vi "MGI RWA Enque Top Level Data.vi"(5 "Format String (%#_13g)":string, 6 "Conversion":T3, 7 "Read/Write Options":T2={"TS Fmt"="", "Int Fmt"="", "Delimiter"=","}, 8 "Error In":errorcluster, 9 "Anything":variant, 10 "Read String":string, 11 "Data Queue In":refnum<queue>) -> (0 "Error Out":errorcluster, 1 "Read State":T1={"StrToSpecifiedText"=variant, "Specified Data"=variant, "Float Fmt"="%#_13g", "Major Vers"=0, "Options"={"TS Fmt"="", "Int Fmt"="", "Delimiter"=","}}, 2 "Tag to String":variant, 3 "Data Queue Our":refnum<queue>, 4 "Warnings":string)   [LabVIEW 2020]
doc: "Add top level data to processing queue. This VI is called both by String to Anything (To Anything=T) and by Anything to String (To Anything=F). Tag to String and Read State are valid only if To Anything=T.\n\nAuthored by Shawn D. Walpole\nsupport@mooregoodideas.com\nwww.mooregoodideas.com\n\nCopyright (c) 2010, Moore Good Ideas, Inc.\n\nAll rights reserved.\n\nRedistribution and use in source and binary forms, with or without modification, are permitted provided that the following conditions are met:\n\n * Redistributions of source code must retain the above copyright notice, this list of conditions and the following disclaimer.\n * Redistributions in binary form must reproduce the above copyright notice, this list of conditions and the following disclaimer in the documentation and/or other materials provided with the distribution.\n * Neither the name of Moore Good Ideas, Inc. nor the names of its contributors may be used to endorse or promote products derived from this software without specific prior written permission.\n\nTHIS SOFTWARE IS PROVIDED BY THE COPYRIGHT HOLDERS AND CONTRIBUTORS \"AS IS\" AND ANY EXPRESS OR IMPLIED WARRANTIES, INCLUDING, BUT NOT LIMITED TO, THE IMPLIED WARRANTIES OF MERCHANTABILITY AND FITNESS FOR A PARTICULAR PURPOSE ARE DISCLAIMED. IN NO EVENT SHALL THE COPYRIGHT OWNER OR CONTRIBUTORS BE LIABLE FOR ANY DIRECT, INDIRECT, INCIDENTAL, SPECIAL, EXEMPLARY, OR CONSEQUENTIAL DAMAGES (INCLUDING, BUT NOT LIMITED TO, PROCUREMENT OF SUBSTITUTE GOODS OR SERVICES; LOSS OF USE, DATA, OR PROFITS; OR BUSINESS INTERRUPTION) HOWEVER CAUSED AND ON ANY THEORY OF LIABILITY, WHETHER IN CONTRACT, STRICT LIABILITY, OR TORT (INCLUDING NEGLIGENCE OR OTHERWISE) ARISING IN ANY WAY OUT OF THE USE OF THIS SOFTWARE, EVEN IF ADVISED OF THE POSSIBILITY OF SUCH DAMAGE."
uses:
  MGI RWA Options Cluster.ctl
  MGI RWA Convertion Direction Enum.ctl
  MGI RWA Tag Lookup Cluster.ctl
  <vilib>/Utility/VariantDataType/Type.ctl
  <vilib>/Utility/VariantDataType/VariantType.lvlib
  String/MGI Windows Get Regional String/MGI Windows Regional Ring.ctl
  <vilib>/Utility/Data Type/NI_Data Type.lvlib
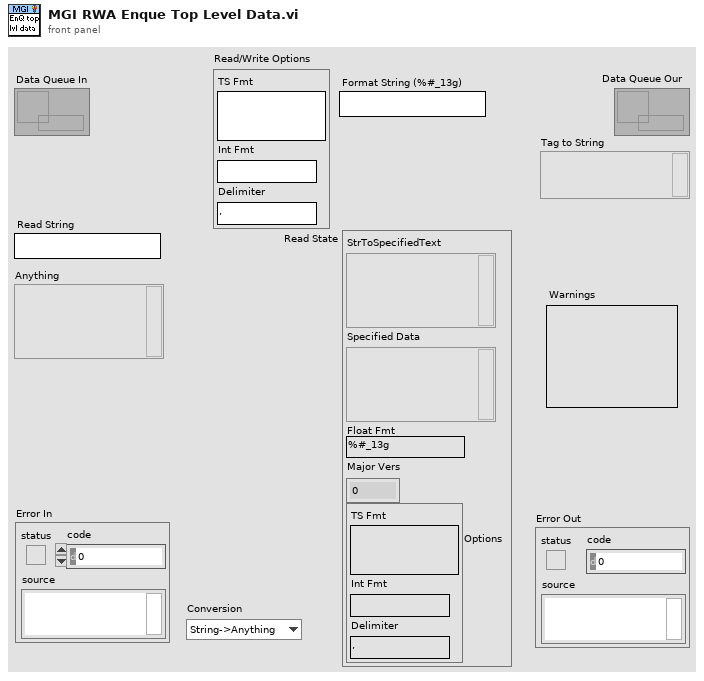
[diagram p1: front panel]
types:
  T1 = typedef "MGI RWA Tag Lookup Cluster.ctl" = cluster{"StrToSpecifiedText":variant, "Specified Data":variant, "Float Fmt":string, "Major Vers":i32, "Options":T2}
  T2 = typedef "MGI RWA Options Cluster.ctl" = cluster{"TS Fmt":string, "Int Fmt":string, "Delimiter":string}
  T3 = typedef "MGI RWA Convertion Direction Enum.ctl" = enum16{"String->Anything", "Anything->String"}
  T4 = typedef "MGI Windows Regional Ring.ctl" = u32
  T5 = typedef "NI_Data Type.lvlib/Data Type.ctl" = enum8{"Invalid Type", "Void", "I8", "I16", "I32", "I64", "U8", "U16", "U32", "U64", "Single Float", "Double Float", "Extended Float", "Single Complex", "Double Complex", "Extended Complex", "Enum U8", "Enum U16", "Enum U32", "Enum U64", "Single Float With Unit", "Double Float With Unit", "Extended Float With Unit", "Single Complex with Unit", "Double Complex with Unit", "Extended Complex with Unit", "Boolean", "String", "Path", "Picture", "Tag", "Array", "Cluster", "Variant", "LV Variant", "Waveform", "Timestamp", "Digital Waveform", "Digital Data", "ExpressData", "Refnum", "External Data", "VI", "Poly VI", "LabVIEW Class Instance", "Fixed Point", "Set Collection", "Map Collection"}
  T6 = typedef "VariantType.lvlib/Type.ctl" = enum8{"Invalid Type", "Void", "I8", "I16", "I32", "I64", "U8", "U16", "U32", "U64", "Single Float", "Double Float", "Extended Float", "Single Complex", "Double Complex", "Extended Complex", "Enum U8", "Enum U16", "Enum U32", "Enum U64", "Single Float With Unit", "Double Float With Unit", "Extended Float With Unit", "Single Complex with Unit", "Double Complex with Unit", "Extended Complex with Unit", "Boolean", "String", "Path", "Picture", "Tag", "Array", "Cluster", "Variant", "LV Variant", "Waveform", "Timestamp", "Digital Waveform", "Digital Data", "ExpressData", "Refnum", "External Data", "VI", "Poly VI", "LabVIEW Class Instance", "Fixed Point"}
  T7 = typedef "NI_Data Type.lvlib/Type Definition Info.ctl" = cluster{"Name":string, "Timestamp":u32}
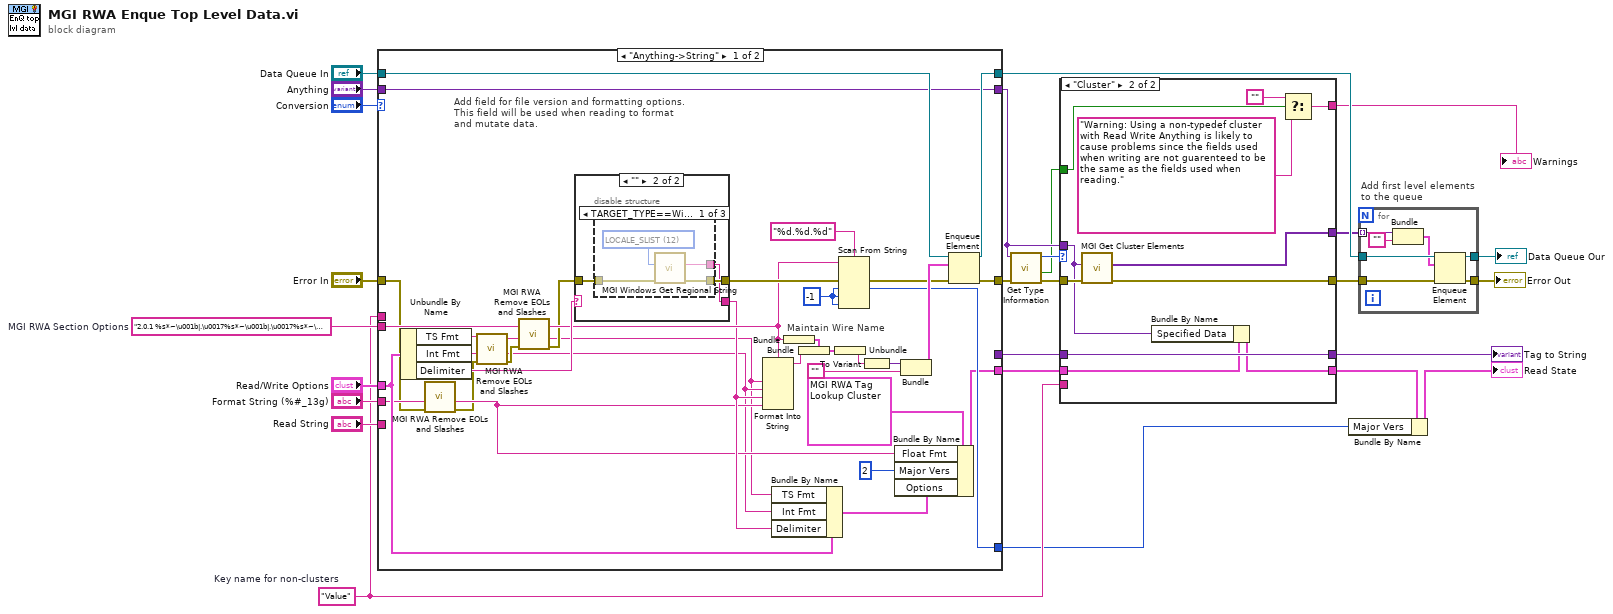
[diagram p0: block diagram]
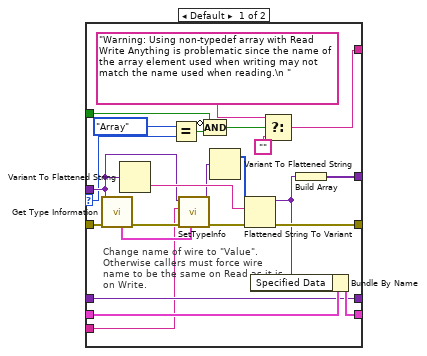
[diagram p2: hidden frame]
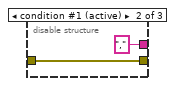
[diagram p4: hidden frame]
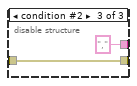
[diagram p5: hidden frame]
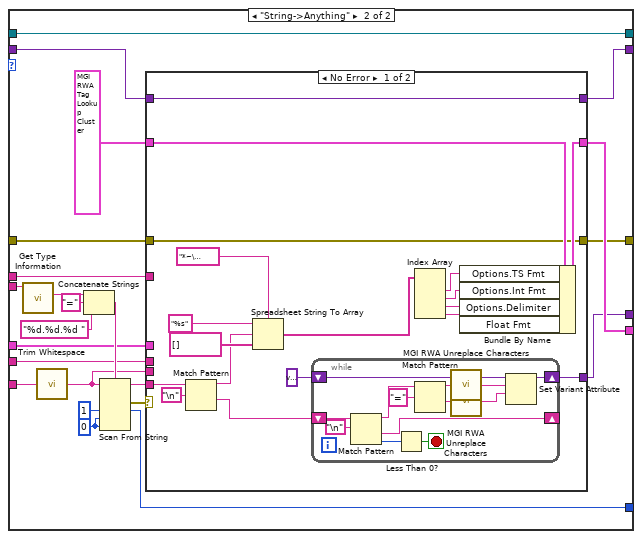
[diagram p6: hidden frame]
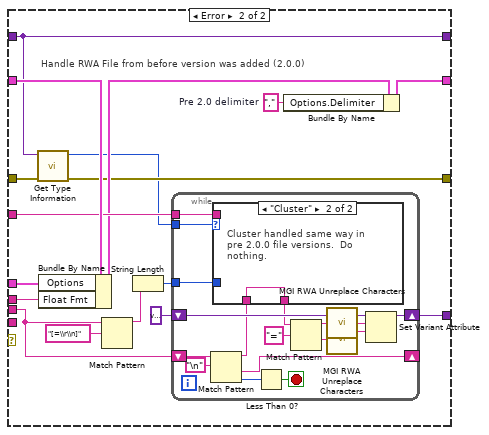
[diagram p7: hidden frame]
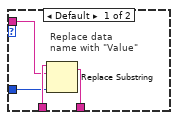
[diagram p8: hidden frame]
diagram:
  w8 = "Value"  # Key name for non-clusters
  w24 = "2.0.1 %s*~\u001b|.\u0017%s*~\u001b|.\u0017%s*~\u001b|.\u0017%s"  # MGI RWA Section Options
  # "Add first level elements\nto the queue"
  n1 = case shown="\"Anything->String\"" "Conversion" {
    tunnel: "Error In" -> [w29 w83]
    tunnel: [w60 w81] -> w13
    tunnel: [w59 w82] -> w26
    tunnel: "Read/Write Options" -> [w40 w86]
    tunnel: w24 -> [w47 w96]
    tunnel: "Data Queue In" -> [w56 w82]
    tunnel: "Format String (%#_13g)" -> [w32 w87]
    tunnel: [w41 w84] -> w10
    tunnel: "Read String" -> [_ w75]
    tunnel: [_ w80] -> w11
    tunnel: [w51 w78] -> w5
    tunnel: w8 -> [_ w79]
    tunnel: "Anything" -> [w48 w77]
    tunnel: [w48 w76] -> w3
    frame "Anything->String" {
      w52 = -1 ("default value 1")
      # "Maintain Wire Name"
      # "Add field for file version and formatting options.  This field will be used when reading to format and mutate data."
      n2 = Unbundle By Name(w40) -> ("TS Fmt"=w34:string, "Int Fmt"=w36:string, "Delimiter"=w49:string)
      n3 = call "MGI RWA Remove EOLs and Slashes.vi"("error in (no error)"=w29, "Format String"=w32) -> ("error out"=w30:errorcluster, "Format String without \\n"=w31:string)  [unwired: 8 in]
      n4 = call "MGI RWA Remove EOLs and Slashes.vi"("error in (no error)"=w30, "Format String"=w36) -> ("error out"=w35:errorcluster, "Format String without \\n"=w28:string)  [unwired: 8 in]
      n5 = call "MGI RWA Remove EOLs and Slashes.vi"("error in (no error)"=w35, "Format String"=w34) -> ("error out"=w33:errorcluster, "Format String without \\n"=w27:string)  [unwired: 8 in]
      n6 = case shown="\"\"" w49 {
        selector: w49 -> [w61 _]
        tunnel: w33 -> [w62 w65]
        tunnel: [w62 w64] -> w50
        tunnel: [w61 w63] -> w39
        frame Default {
        }
        frame "" {
          n7 = disable-structure shown="TARGET_TYPE==Windows" {
            disable-tunnel: [w68 "," ("List Seperator") "," ("List Seperator")] -> w63
            disable-tunnel: w65 -> [w67 w70 w73]
            disable-tunnel: [w66 w70 w73] -> w64
            frame condition #0 {
              w69 = T4 12 items=["LOCALE_ILANGUAGE"=1, "LOCALE_SLANGUAGE"=2, "LOCALE_SABBREVLANGNAME"=3, "LOCALE_SNATIVELANGNAME"=4, "LOCALE_ICOUNTRY"=5, "LOCALE_SCOUNTRY"=6, "LOCALE_SABBREVCTRYNAME"=7, "LOCALE_SNATIVECTRYNAME"=8, "LOCALE_IDEFAULTLANGUAGE"=9, "LOCALE_IDEFAULTCOUNTRY"=10, "LOCALE_IDEFAULTCODEPAGE"=11, "LOCALE_SLIST"=12, "LOCALE_IMEASURE"=13, "LOCALE_SDECIMAL"=14, "LOCALE_STHOUSAND"=15, "LOCALE_SGROUPING"=16, "LOCALE_IDIGITS"=17, "LOCALE_ILZERO"=18, "LOCALE_SNATIVEDIGITS"=19, "LOCALE_SCURRENCY"=20, "LOCALE_SINTLSYMBOL"=21, "LOCALE_SMONDECIMALSEP"=22, "LOCALE_SMONTHOUSANDSEP"=23, "LOCALE_SMONGROUPING"=24, "LOCALE_ICURRDIGITS"=25, "LOCALE_IINTLCURRDIGITS"=26, "LOCALE_ICURRENCY"=27, "LOCALE_INEGCURR"=28, "LOCALE_SDATE"=29, "LOCALE_STIME"=30, "LOCALE_SSHORTDATE"=31, "LOCALE_SLONGDATE"=32, "LOCALE_IDATE"=33, "LOCALE_ILDATE"=34, "LOCALE_ITIME"=35, "LOCALE_ICENTURY"=36, "LOCALE_ITLZERO"=37, "LOCALE_IDAYLZERO"=38, "LOCALE_IMONLZERO"=39, "LOCALE_S1159"=40, "LOCALE_S2359"=41, "LOCALE_SDAYNAME1"=42, "LOCALE_SDAYNAME2"=43, "LOCALE_SDAYNAME3"=44, "LOCALE_SDAYNAME4"=45, "LOCALE_SDAYNAME5"=46, "LOCALE_SDAYNAME6"=47, "LOCALE_SDAYNAME7"=48, "LOCALE_SABBREVDAYNAME1"=49, "LOCALE_SABBREVDAYNAME2"=51, "LOCALE_SABBREVDAYNAME3"=52, "LOCALE_SABBREVDAYNAME4"=53, "LOCALE_SABBREVDAYNAME5"=54, "LOCALE_SABBREVDAYNAME6"=55, "LOCALE_SABBREVDAYNAME7"=56, "LOCALE_SMONTHNAME1"=57, "LOCALE_SMONTHNAME2"=58, "LOCALE_SMONTHNAME3"=59, "LOCALE_SMONTHNAME4"=60, "LOCALE_SMONTHNAME5"=61, "LOCALE_SMONTHNAME6"=62, "LOCALE_SMONTHNAME7"=63, "LOCALE_SMONTHNAME8"=64, "LOCALE_SMONTHNAME9"=65, "LOCALE_SMONTHNAME10"=66, "LOCALE_SMONTHNAME11"=67, "LOCALE_SMONTHNAME12"=68, "LOCALE_SABBREVMONTHNAME1"=69, "LOCALE_SABBREVMONTHNAME2"=70, "LOCALE_SABBREVMONTHNAME3"=71, "LOCALE_SABBREVMONTHNAME4"=72, "LOCALE_SABBREVMONTHNAME5"=73, "LOCALE_SABBREVMONTHNAME6"=74, "LOCALE_SABBREVMONTHNAME7"=75, "LOCALE_SABBREVMONTHNAME8"=76, "LOCALE_SABBREVMONTHNAME9"=77, "LOCALE_SABBREVMONTHNAME10"=78, "LOCALE_SABBREVMONTHNAME11"=79, "LOCALE_SABBREVMONTHNAME12"=80, "LOCALE_SENGLANGUAGE"=4097, "LOCALE_SENGCOUNTRY"=4098, "LOCALE_STIMEFORMAT"=4099, "LOCALE_SABBREVMONTHNAME13"=4111] ("Regional Item")
              n8 = call "MGI Windows Get Regional String.vi"("error in (no error)"=w67, "Regional Item"=w69) -> ("error out"=w66:errorcluster, "List Seperator"=w68:string)  [unwired: 8 in]
            }
            frame condition #1 (active) {
            }
            frame condition #2 {
            }
          }
        }
      }
      n9 = Format Into String(format string=w47, w27, w28, w39, w31) -> (resulting string=w46:string)  [unwired: 2 in, 1 out]
      n10 = Bundle By Name(cluster=w40, "TS Fmt"=w27, "Int Fmt"=w28, "Delimiter"=w39) -> (w38:T2)
      n11 = Bundle("MGI RWA Section Options"=w47) -> (w45:cluster{"MGI RWA Section Options":string})  [unwired: 1 in]
      n12 = Bundle(cluster=w45, "MGI RWA Section Options"=w46) -> (w44:cluster{"MGI RWA Section Options":string})
      n13 = Unbundle(w44) -> ("MGI RWA Section Options"=w43:string)
      n14 = Scan From String(format string="%d.%d.%d", input string=w47, error in=w50, default 1=w52, default 2=w52, default 3=w52) -> (error out=w54:errorcluster, output 1=w51:i32)  [unwired: 3 in, 2 out]
      n15 = To Variant(anything=w43) -> (Variant=w55:variant)
      n16 = Bundle By Name(cluster=T1 {"StrToSpecifiedText"=variant, "Specified Data"=variant, "Float Fmt"="", "Major Vers"=0, "Options"={"TS Fmt"="", "Int Fmt"="", "Delimiter"=""}} ("State In"), "Float Fmt"=w31, "Major Vers"=2, "Options"=w38) -> (w41:T1)
      n17 = Bundle("Variant"=w55, "") -> (w57:cluster{"Variant":variant, string})  [unwired: 1 in]
      n18 = Enqueue Element(queue=w56, element=w57, error in (no error)=w54) -> (queue out=w59:refnum<queue>, error out=w60:errorcluster)  [unwired: 1 in, 1 out]
    }
    frame "String->Anything" {
      w92 = 0 ("default value 1")
      n19 = call <vilib>:"Get Type Information.vi"("variant"=w96) -> ("name"=w95:string)  [unwired: 6 in, 4 out]
      n20 = call <vilib>:"Trim Whitespace.vi"("string"=w75) -> ("trimmed string"=w74:string)  [unwired: 1 in]
      n21 = Concatenate Strings(w95, "=" ("string"), "%d.%d.%d ") -> (w90:string)
      n22 = Scan From String(format string=w90, input string=w74, default 1=1 ("default value 1"), default 2=w92, default 3=w92) -> (remaining string=w88:string, error out=w89:errorcluster, output 1=w78:i32)  [unwired: 4 in, 1 out]
      n23 = case shown="No Error" w89 {
        tunnel: w88 -> [w113 _]
        tunnel: w87 -> [_ w143]
        tunnel: w86 -> [_ w136]
        tunnel: T1 {"StrToSpecifiedText"=variant, "Specified Data"=variant, "Float Fmt"="", "Major Vers"=0, "Options"={"TS Fmt"="", "Int Fmt"="", "Delimiter"=""}} ("State In") -> [w108 w144]
        tunnel: [w107 w134] -> w84
        tunnel: w83 -> [w97 w132]
        tunnel: [w97 w131] -> w81
        tunnel: [w101 w141] -> w80
        tunnel: w79 -> [_ w139]
        tunnel: w77 -> [w98 w130]
        tunnel: [w98 w130] -> w76
        tunnel: w74 -> [_ w128]
        frame No Error {
          n24 = Match Pattern(string=w113, regular expression="\n") -> (before substring=w109:string, after substring=w102:string)  [unwired: 1 in, 2 out]
          n25 = Spreadsheet String To Array(delimiter (Tab)="*~\u001b|.\u0017", format string="%s", spreadsheet string=w109, array type (2D Dbl)=string[] []) -> (array=w106:string[])
          n26 = while {
            shift-right: [w125] -> _
            shift-left: w102 -> [w127]
            shift-right: [w120] -> w101
            shift-left: variant ("variant") -> [w121]
            stop <- w123 stop-if-true
            n27 = Match Pattern(string=w127, regular expression="\n") -> (before substring=w119:string, after substring=w125:string, offset past match=w124:i32)  [unwired: 1 in, 1 out]
            n28 = Less Than 0?(x=w124) -> (x < 0?=w123:bool)
            n29 = Match Pattern(string=w119, regular expression="=") -> (before substring=w118:string, after substring=w117:string)  [unwired: 1 in, 2 out]
            n30 = call "MGI RWA Unreplace Characters.vi"("String In"=w118) -> ("String Out"=w116:string)  [unwired: 1 in]
            n31 = call "MGI RWA Unreplace Characters.vi"("String In"=w117) -> ("String Out"=w115:string)  [unwired: 1 in]
            n32 = Set Variant Attribute(Variant=w121, name=w116, value=w115) -> (Variant out=w120:variant)  [unwired: 1 in, 2 out]
          }
          n33 = Index Array(array=w106) -> (element #1=w105:string, element #2=w104:string, element #3=w100:string, element #4=w99:string)  [unwired: 4 in]
          n34 = Bundle By Name(cluster=w108, "Options.TS Fmt"=w105, "Options.Int Fmt"=w104, "Options.Delimiter"=w100, "Float Fmt"=w99) -> (w107:T1)
        }
        frame Error {
          w133 = ","  # Pre 2.0 delimiter
          # "Handle RWA File from before version was added (2.0.0)"
          n35 = call <vilib>:"Get Type Information.vi"("error in (no error)"=w132, "variant"=w130) -> ("error out"=w131:errorcluster, "type"=w129:T5)  [unwired: 5 in, 3 out]
          n36 = Bundle By Name(cluster=w144, "Options"=w136, "Float Fmt"=w143) -> (w135:T1)
          n37 = Match Pattern(string=w128, regular expression="[=\\r\\n]") -> (before substring=w138:string)  [unwired: 1 in, 3 out]
          n38 = String Length(string=w138) -> (length=w137:i32)
          n39 = while {
            shift-right: [w159] -> _
            shift-left: w128 -> [w161]
            shift-right: [w154] -> w141
            shift-left: variant ("variant") -> [w155]
            tunnel: w129 -> [w149]
            tunnel: w137 -> [w146]
            tunnel: w139 -> [w145]
            stop <- w157 stop-if-true
            n40 = Match Pattern(string=w161, regular expression="\n") -> (before substring=w148:string, after substring=w159:string, offset past match=w158:i32)  [unwired: 1 in, 1 out]
            n41 = case shown="\"Cluster\"" w149 {
              tunnel: w148 -> [w165 w166]
              tunnel: [w163 w166] -> w147
              tunnel: w146 -> [w162 _]
              tunnel: w145 -> [w164 _]
              frame Default {
                # "Replace data name with \"Value\""
                n42 = Replace Substring(2:w162, 4:w164, 5:w165) -> (1:w163:string)  [unwired: 1 in, 1 out]
              }
              frame "Cluster" {
                # "Cluster handled same way in pre 2.0.0 file versions.  Do nothing."
              }
            }
            n43 = Less Than 0?(x=w158) -> (x < 0?=w157:bool)
            n44 = Match Pattern(string=w147, regular expression="=") -> (before substring=w153:string, after substring=w152:string)  [unwired: 1 in, 2 out]
            n45 = call "MGI RWA Unreplace Characters.vi"("String In"=w153) -> ("String Out"=w151:string)  [unwired: 1 in]
            n46 = call "MGI RWA Unreplace Characters.vi"("String In"=w152) -> ("String Out"=w150:string)  [unwired: 1 in]
            n47 = Set Variant Attribute(Variant=w155, name=w151, value=w150) -> (Variant out=w154:variant)  [unwired: 1 in, 2 out]
          }
          n48 = Bundle By Name(cluster=w135, "Options.Delimiter"=w133) -> (w134:T1)
        }
      }
    }
  }
  n49 = call <vilib>:"Get Type Information.vi"("error in (no error)"=w13, "variant"=w3) -> ("error out"=w15:errorcluster, "type definition"=w2:bool, "type"=w16:T5)  [unwired: 5 in, 2 out]
  n50 = case shown="\"Cluster\"" w16 {
    selector: w16 -> [w174 _]
    tunnel: [w176 w200] -> w12
    tunnel: w3 -> [w181 w194]
    tunnel: w15 -> [w182 w199]
    tunnel: [w183 w198] -> w14
    tunnel: w11 -> [w178 w197]
    tunnel: w10 -> [w180 w196]
    tunnel: [w178 w197] -> w9
    tunnel: [w179 w195] -> w7
    tunnel: w8 -> [w175 _]
    tunnel: w2 -> [w171 w193]
    tunnel: [w167 w190] -> w1
    frame Default {
      # "Change name of wire to \"Value\".\nOtherwise callers must force wire name to be the same on Read as it is on Write."
      n51 = call <vilib>:"Get Type Information.vi"("error in (no error)"=w182, "variant"=w181) -> ("error out"=w184:errorcluster, "type definition info"=w185:T7)  [unwired: 5 in, 3 out]
      n52 = Variant To Flattened String(Variant=w181) -> (data string=w188:string)  [unwired: 1 out]
      n53 = Equal?(x=Type."Array", y=w174) -> (x = y?=w170:bool)
      n54 = call <vilib>:"SetTypeInfo.vi"("Typedef Info"=w185, "error in (no error)"=w184, "Name"=w175, "Variant"=w181) -> ("error out"=w189:errorcluster, "Variant Out"=w186:variant)  [unwired: 6 in]
      n55 = Compound Arithmetic op=AND(invert w171, w170) -> (w169:bool)
      n56 = Variant To Flattened String(Variant=w186) -> (1:w187:i16[])  [unwired: 1 out]
      n57 = Flattened String To Variant(4:w189, 6:w188, 7:w187) -> (0:w183:errorcluster, 3:w177:variant)
      n58 = Bundle By Name(cluster=w180, "Specified Data"=w177) -> (w179:T1)
      n59 = Select(t="Warning: Using non-typedef array with Read Write Anything is problematic since the name of the array element used when writing may not match the name used when reading.\n ", s=w169, f="") -> (s? t:f=w167:string)
      n60 = Build Array(w177) -> (w176:variant[])
    }
    frame "Cluster" {
      n61 = call "MGI Get Cluster Elements.vi"("Error In"=w199, "Cluster"=w194) -> ("Error Out"=w198:errorcluster, "Cluster Elements"=w200:variant[])  [unwired: 8 in]
      n62 = Bundle By Name(cluster=w196, "Specified Data"=w194) -> (w195:T1)
      n63 = Select(t="", s=w193, f="Warning: Using a non-typedef cluster with Read Write Anything is likely to cause problems since the fields used when writing are not guarenteed to be the same as the fields used when reading.") -> (s? t:f=w190:string)
    }
  }
  "Tag to String" <- w9
  "Warnings" <- w1
  n64 = Bundle By Name(cluster=w7, "Major Vers"=w5) -> (→"Read State":T1)
  n65 = for {
    tunnel: w26 -> [w207]
    tunnel: w14 -> [w206]
    tunnel: [w205] -> w20
    tunnel: [w204] -> w22
    tunnel: w12 -> [w202] mode=indexing
    n66 = Bundle("Variant"=w202, "") -> (w203:cluster{"Variant":variant, string})  [unwired: 1 in]
    n67 = Enqueue Element(queue=w207, element=w203, error in (no error)=w206) -> (queue out=w204:refnum<queue>, error out=w205:errorcluster)  [unwired: 1 in, 1 out]
  }
  "Error Out" <- w20
  "Data Queue Our" <- w22
